vi "CDW_SpecPage.vi"(10 "Spec Page Interface":T2, 11 "MetaDataObj in":refnum<class "MetaDataObj.lvclass">) -> (3 "MetaDataObj out":refnum<class "MetaDataObj.lvclass">)   [LabVIEW 2015, in "NIVS_Consolidated_CDW_MetaDataObj.lvclass"]
uses:
  NIVS_Consolidated_CDW_MetaDataObj.lvclass
  <resource>/dialog/NewProjectWizard/Spec Page Interface.ctl
  <resource>/dialog/NewProjectWizard/MetaDataObj/MetaDataObj.lvclass
  Template Classes/NIVS_Asynchronous/NIVS_Asynchronous.lvclass
  Template Classes/NIVS_Inline HW Interface (Inline-Async)/NIVS_Inline HW Interface (Inline-Async).lvclass
  Template Classes/NIVS_Inline HW Interface/NIVS_Inline HW Interface.lvclass
  Template Classes/NIVS_Inline Model Interface/NIVS_Inline Model Interface.lvclass
  Template Classes/NIVS_Inline Timing and Sync/NIVS_Inline Timing and Sync.lvclass
  Template Classes/NIVS_Asynchronous Timing and Sync/NIVS_Asynchronous Timing and Sync.lvclass
  Template Classes/NIVS_CD Template/NIVS_CD Template.lvclass/NIVS_CD Template.ctl
  NIVS_Consolidated_CDW_MetaDataObj.lvclass/NIVS_Consolidated_CDW_MetaDataObj.ctl
  <resource>/dialog/NewProjectWizard/MetaDataObj/MetaDataObj.lvclass/MetaDataObj.ctl
  Execution Mode.ctl
  Template Classes/NIVS_CD Template/Write Max Instances.vi
  Template Classes/NIVS_CD Template/Write Extra Page Names.vi
  Template Classes/NIVS_CD Template/Write Submenu.vi
  Template Classes/NIVS_CD Template/Write Parent Menu.vi
  <resource>/dialog/NewProjectWizard/MetaDataObj/Accessors/Write Project Name.vi
  <resource>/dialog/NewProjectWizard/MetaDataObj/Accessors/Write Project Root.vi
  Template Classes/NIVS_CD Template/NIVS_CD Template.lvclass
panel:
  in  "Inline-Async":bool=TRUE
  in  "Custom Device Execution Mode":T1(ring)=enum."Inline HW Interface"
  in  "Custom Device Name":string
  in  "Project Root":path
  in  "Maximum Custom Device Instances":u32=1 min=1 max=2474 step=1
  in  "Insert Custom Device in submenu":bool
  in  "Parent Menu Name":string
  in  "Custom Device Extra Page Names":string[](array[string])
  # "Advanced Options"
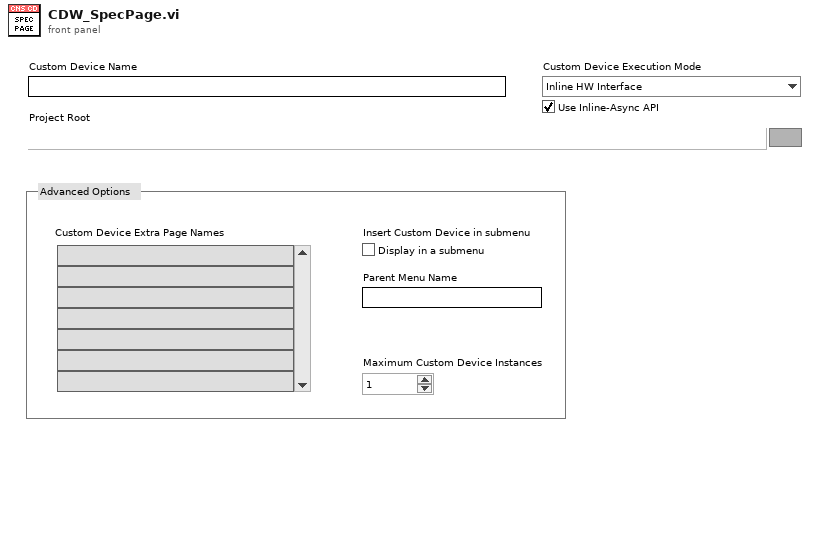
[diagram p1: front panel]
types:
  T1 = enum16{"Asynchronous", "Inline HW Interface", "Inline Model Interface", "Inline Timing and Sync", "Asynchronous Timing and Sync"}
  T2 = typedef "Spec Page Interface.ctl" = cluster{"\"Tab Forward To\" Refnum":refnum<vi>, "\"Tab Backward To\" Refnum":refnum<vi>, "Errors":refnum<user-event>, "Quit":refnum<user-event>}
  T3 = enum8{"Enabled", "Disabled", "Disabled and Grayed Out"}
  T4 = typedef "NIVS_Consolidated_CDW_MetaDataObj.lvclass/Execution Mode.ctl" = enum16{"Asynchronous", "Inline HW Interface", "Inline Model Interface", "Inline Timing and Sync", "Asynchronous Timing and Sync"}
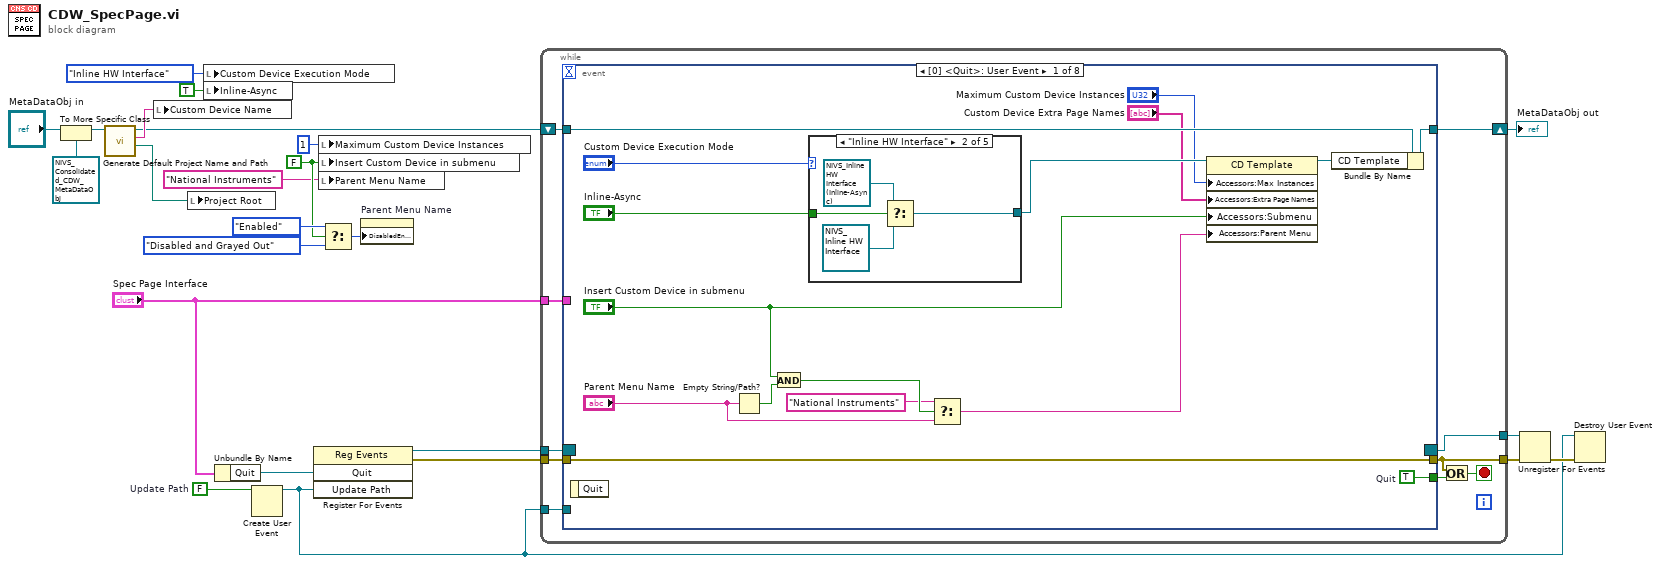
[diagram p0: block diagram]
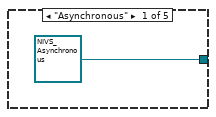
[diagram p2: hidden frame]
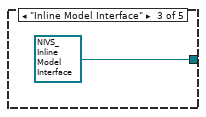
[diagram p3: hidden frame]
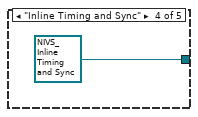
[diagram p4: hidden frame]
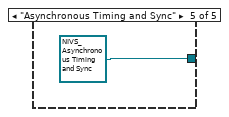
[diagram p5: hidden frame]
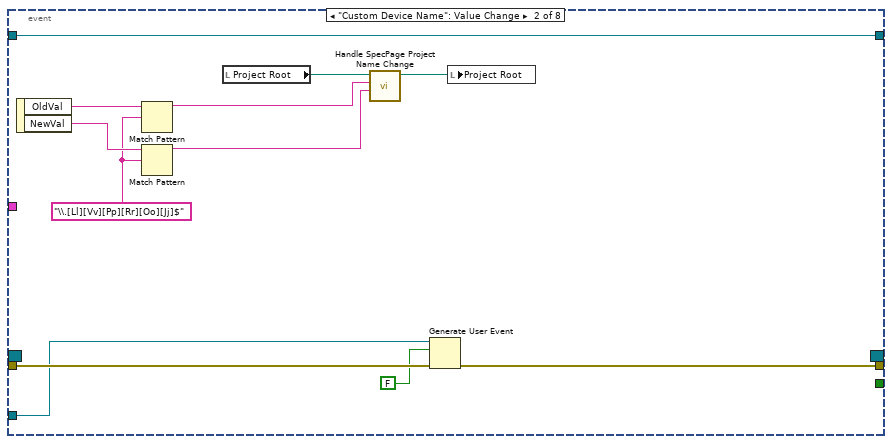
[diagram p6: hidden frame]
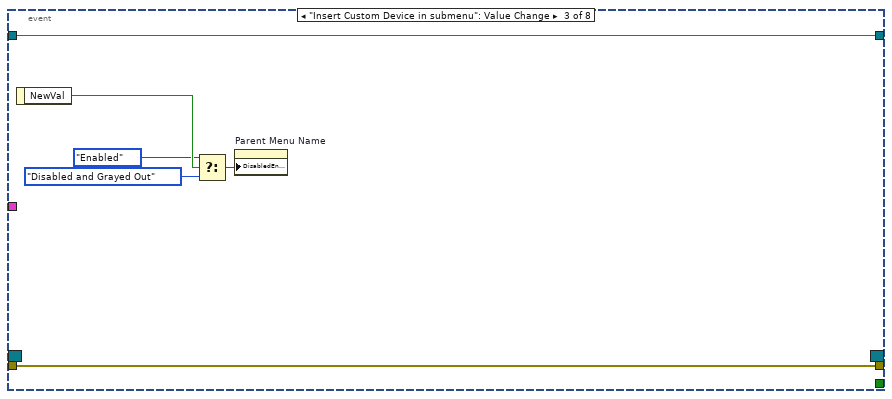
[diagram p7: hidden frame]
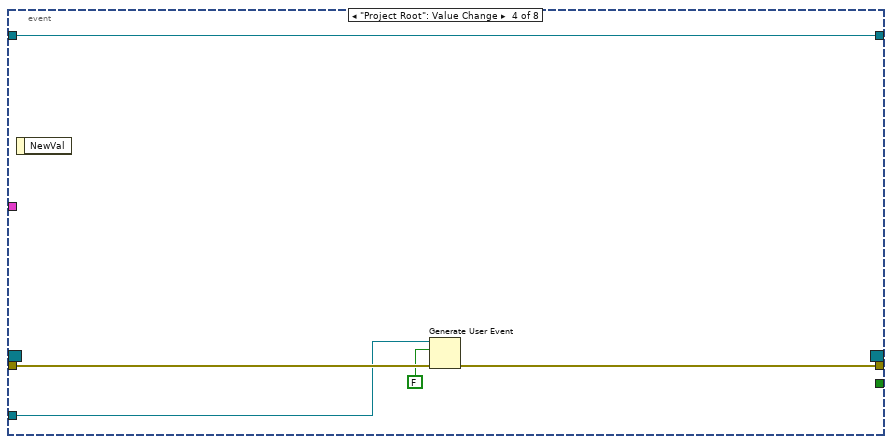
[diagram p8: hidden frame]
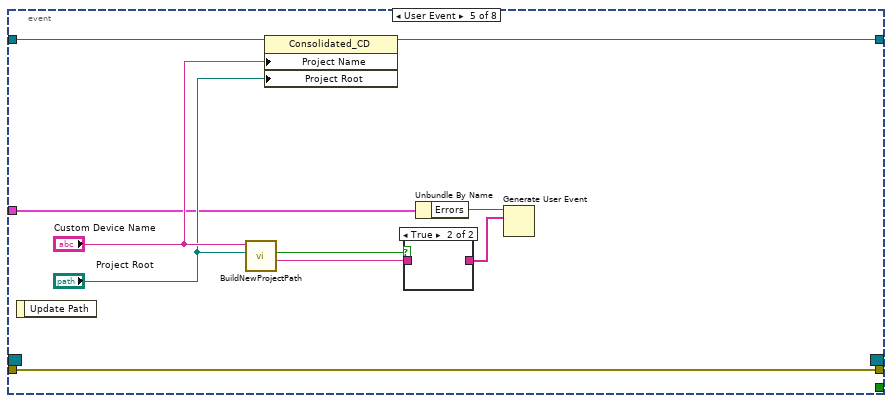
[diagram p9: hidden frame]
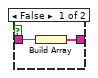
[diagram p10: hidden frame]
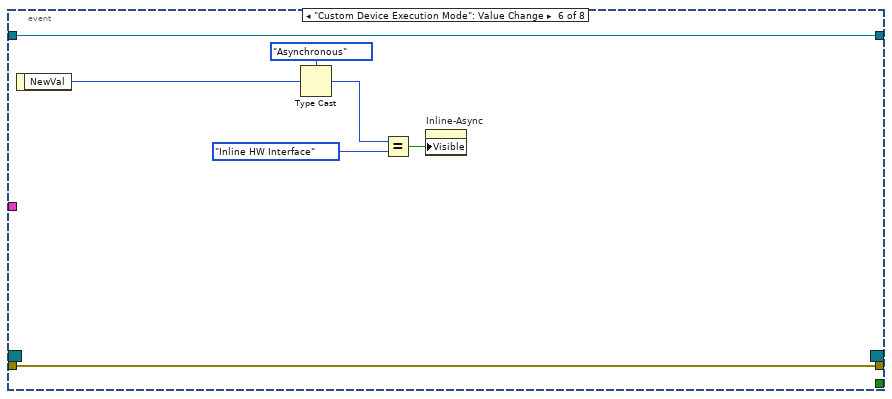
[diagram p11: hidden frame]
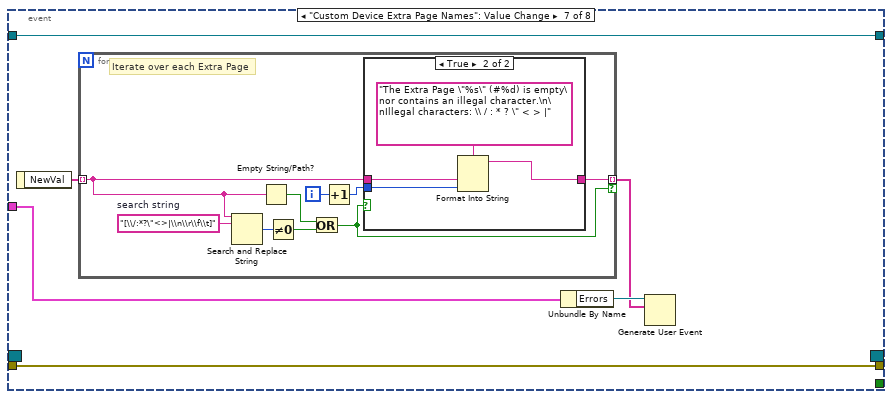
[diagram p12: hidden frame]
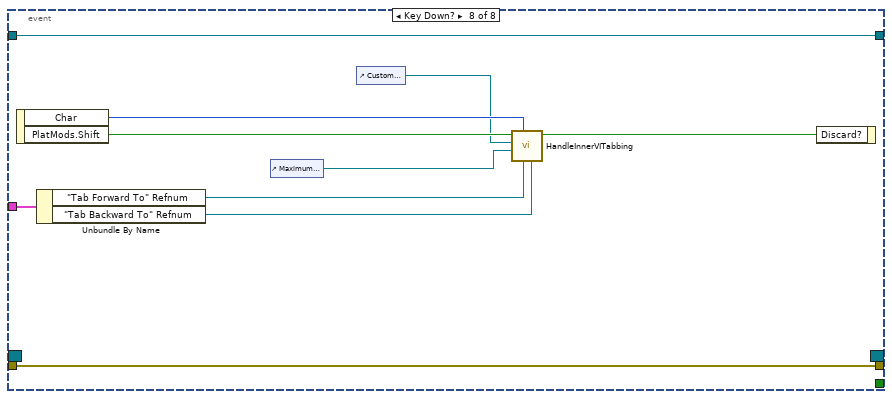
[diagram p14: hidden frame]
diagram:
  w5 = FALSE
  w8 = FALSE  # Update Path
  n1 = To More Specific Class(target class=refnum<class "NIVS_Consolidated_CDW_MetaDataObj.lvclass"> refnum ("Consolidated"), reference="MetaDataObj in") -> (specific class reference=w11:refnum<class "NIVS_Consolidated_CDW_MetaDataObj.lvclass">)  [unwired: 1 in, 1 out]
  n2 = call <resource>:"Generate Default Project Name and Path.vi"("DNL_MetaDataObj in"=w11) -> ("Project Root"=w9:path, "Project Name"=w14:string, "DNL_MetaDataObj out"=w10:refnum<class "NIVS_Consolidated_CDW_MetaDataObj.lvclass">)  [unwired: 8 in]
  n3 = local write "Custom Device Name"(w14) -> ()
  n4 = local write "Project Root"(w9) -> ()
  n5 = local write "Custom Device Execution Mode"(T1."Inline HW Interface" ("Custom Device Execution Mode")) -> ()
  n6 = local write "Inline-Async"(TRUE ("Inline-Async")) -> ()
  n7 = Unbundle By Name("Spec Page Interface") -> ("Quit"=w24:refnum<user-event>)
  n8 = Create User Event(user event datatype=w8) -> (user event=w6:refnum<user-event>)  [unwired: 1 in, 1 out]
  n9 = register-events(w24, w6) -> (reference out=w23:refnum<event-registration>, error out=w19:errorcluster)  [unwired: 2 in]
  n10 = local write "Maximum Custom Device Instances"(u32 1 ("Maximum Custom Device Instances")) -> ()
  n11 = local write "Insert Custom Device in submenu"(w5) -> ()
  n12 = local write "Parent Menu Name"("National Instruments") -> ()
  n13 = Select(t=T3."Enabled" ("Disabled"), s=w5, f=T3."Disabled and Grayed Out") -> (s? t:f=w17:T3)
  n14 = property on="Parent Menu Name" class="Str"("DisabledEnum"=w17) -> ()  [unwired: 2 in, 2 out]
  n15 = while {
    tunnel: "Spec Page Interface" -> [w32]
    shift-right: [w31] -> w20
    shift-left: w10 -> [w30]
    tunnel: w23 -> [w34]
    tunnel: w19 -> [w33]
    tunnel: [w27] -> w21
    tunnel: [w26] -> w13
    tunnel: w6 -> [w25]
    stop <- w29 stop-if-true
    n16 = event shown="[0] <Quit>: User Event" {
      selector: w34 -> [_ _ _ _ _ _ _ _]
      dyn-events: [_ _ _ _ _ _ _ _] -> w26
      timeout: _ -> [_ _ _ _ _ _ _ _]
      tunnel: w32 -> [_ _ _ _ w86 _ w102 w125]
      tunnel: [w50 _ _ _ _ _ _ _] -> w28
      tunnel: [w49 w61 w76 w79 w91 w100 w106 w130] -> w27
      tunnel: w33 -> [w49 w70 w76 w81 w91 w100 w106 w130]
      tunnel: [w47 w69 w75 w80 w89 w99 w104 w129] -> w31
      tunnel: w30 -> [w48 w69 w75 w80 w90 w99 w104 w129]
      tunnel: w25 -> [_ w60 _ w78 _ _ _ _]
      event User Event {
        w50 = TRUE  # Quit
        n17 = event-data() -> ()  [unwired: 1 in, 1 out]
        n18 = Empty String/Path?(string/path="Parent Menu Name") -> (empty?=w45:bool)
        n19 = And(x="Insert Custom Device in submenu", y=w45) -> (x .and. y?=w44:bool)
        n20 = case shown="\"Inline HW Interface\"" "Custom Device Execution Mode" {
          tunnel: "Inline-Async" -> [_ w55 _ _ _]
          tunnel: [refnum<class "NIVS_Asynchronous.lvclass"> refnum ("NIVS_Asynchronous.lvclass") w52 refnum<class "NIVS_Inline Model Interface.lvclass"> refnum ("NIVS_Inline Model Interface.lvclass") refnum<class "NIVS_Inline Timing and Sync.lvclass"> refnum ("NIVS_Inline Timing and Sync.lvclass") refnum<class "NIVS_Asynchronous Timing and Sync.lvclass"> refnum ("NIVS_Asynchronous Timing and Sync.lvclass")] -> w39
          frame "Asynchronous" {
          }
          frame "Inline HW Interface" {
            n21 = Select(t=refnum<class "NIVS_Inline HW Interface (Inline-Async).lvclass"> refnum ("NIVS_Inline HW Interface (Inline-Async).lvclass"), s=w55, f=refnum<class "NIVS_Inline HW Interface.lvclass"> refnum ("NIVS_Inline HW Interface.lvclass")) -> (s? t:f=w52:refnum<class "NIVS_CD Template.lvclass">)
          }
          frame "Inline Model Interface" {
          }
          frame "Inline Timing and Sync" {
          }
          frame "Asynchronous Timing and Sync" {
          }
        }
        n22 = Select(t="National Instruments", s=w44, f="Parent Menu Name") -> (s? t:f=w35:string)
        n23 = property class="CD Template"(reference=w39, "Accessors:Max Instances"="Maximum Custom Device Instances", "Accessors:Extra Page Names"="Custom Device Extra Page Names", "Accessors:Submenu"="Insert Custom Device in submenu", "Accessors:Parent Menu"=w35) -> (reference out=w40:refnum<class "NIVS_CD Template.lvclass">)  [unwired: 1 in, 1 out]
        n24 = Bundle By Name(cluster=w48, "CD Template"=w40) -> (w47:refnum<class "NIVS_Consolidated_CDW_MetaDataObj.lvclass">)
      }
      event "Custom Device Name": Value Change {
        w66 = "\\.[Ll][Vv][Pp][Rr][Oo][Jj]$"
        n25 = event-data() -> ("OldVal"=w68:string, "NewVal"=w67:string)  [unwired: 1 in]
        n26 = Match Pattern(string=w68, regular expression=w66) -> (before substring=w63:string)  [unwired: 1 in, 3 out]
        n27 = Match Pattern(string=w67, regular expression=w66) -> (before substring=w62:string)  [unwired: 1 in, 3 out]
        n28 = local read "Project Root"() -> (w65:path)
        n29 = call <resource>:"Handle SpecPage Project Name Change.vi"("Project Name New Value"=w62, "Project Name Old Value"=w63, "Project Root in"=w65) -> ("Project Root out"=w64:path)  [unwired: 8 in]
        n30 = Generate User Event(user event=w60, event data cluster=FALSE, error in=w70) -> (error out=w61:errorcluster)  [unwired: 1 in, 1 out]
        n31 = local write "Project Root"(w64) -> ()
      }
      event "Insert Custom Device in submenu": Value Change {
        n32 = event-data() -> ("NewVal"=w74:bool)  [unwired: 1 in]
        n33 = Select(t=T3."Enabled" ("Disabled"), s=w74, f=T3."Disabled and Grayed Out") -> (s? t:f=w71:T3)
        n34 = property on="Parent Menu Name" class="Str"("DisabledEnum"=w71) -> ()  [unwired: 2 in, 2 out]
      }
      event "Project Root": Value Change {
        n35 = event-data() -> ()  [unwired: 1 in, 1 out]
        n36 = Generate User Event(user event=w78, event data cluster=FALSE, error in=w81) -> (error out=w79:errorcluster)  [unwired: 1 in, 1 out]
      }
      event User Event {
        n37 = event-data() -> ()  [unwired: 1 in, 1 out]
        n38 = call <resource>:"BuildNewProjectPath.vi"("Project Root"="Project Root", "Project Name"="Custom Device Name") -> ("Error Message"=w85:string, "Valid?"=w82:bool)  [unwired: 7 in, 1 out]
        n39 = property class="Consolidated_CD"(reference=w90, "Project Name"="Custom Device Name", "Project Root"="Project Root") -> (reference out=w89:refnum<class "NIVS_Consolidated_CDW_MetaDataObj.lvclass">)  [unwired: 1 in, 1 out]
        n40 = case shown="True" w82 {
          tunnel: w85 -> [w93 _]
          tunnel: [w92 _] -> w83
          frame False {
            n41 = Build Array(w93) -> (w92:string[])
          }
          frame True {
          }
        }
        n42 = Unbundle By Name(w86) -> ("Errors"=w84:refnum<user-event>)
        n43 = Generate User Event(user event=w84, event data cluster=w83) -> ()  [unwired: 2 in, 2 out]
      }
      event "Custom Device Execution Mode": Value Change {
        n44 = event-data() -> ("NewVal"=w98:T1)  [unwired: 1 in]
        n45 = Type Cast(type=Execution_Mode."Asynchronous" ("CD Wizard - Internal Data.Common Information.CD Execution Mode"), x=w98) -> (*(type *) &x=w96:T4)
        n46 = Equal?(x=w96, y=Execution_Mode."Inline HW Interface") -> (x = y?=w94:bool)
        n47 = property on="Inline-Async" class="Bool (strict)"("Visible"=w94) -> ()  [unwired: 2 in, 2 out]
      }
      event "Custom Device Extra Page Names": Value Change {
        n48 = event-data() -> ("NewVal"=w105:string[])  [unwired: 1 in]
        n49 = for {
          tunnel: w105 -> [w109] mode=indexing
          tunnel: [w108] -> w101 mode=indexing if=w107
          i -> [w111]
          w115 = "[\\/:*?\"<>|\\n\\r\\f\\t]"  # search string
          # "Iterate over each Extra Page"
          n50 = Search and Replace String(input string=w109, search string=w115) -> (number of replacements=w114:i32)  [unwired: 6 in, 3 out]
          n51 = Empty String/Path?(string/path=w109) -> (empty?=w113:bool)
          n52 = Not Equal To 0?(x=w114) -> (x != 0?=w112:bool)
          n53 = Or(x=w113, y=w112) -> (x .or. y?=w107:bool)
          n54 = Increment(x=w111) -> (x+1=w110:i32)
          n55 = case shown="True" w107 {
            tunnel: w110 -> [_ w118]
            tunnel: w109 -> [w116 w119]
            tunnel: [w116 w117] -> w108
            frame False {
              # "Extra Page Name is OK"
            }
            frame True {
              n56 = Format Into String(format string="The Extra Page \"%s\" (#%d) is empty\nor contains an illegal character.\n\nIllegal characters: \\ / : * ? \" < > |", w119, w118) -> (resulting string=w117:string)  [unwired: 2 in, 1 out]
            }
          }
        }
        n57 = Unbundle By Name(w102) -> ("Errors"=w103:refnum<user-event>)
        n58 = Generate User Event(user event=w103, event data cluster=w101) -> ()  [unwired: 2 in, 2 out]
      }
      event Key Down? {
        n59 = event-data() -> ("Char"=w128:i16, "PlatMods.Shift"=w127:bool)  [unwired: 1 in]
        n60 = Unbundle By Name(w125) -> ("\"Tab Forward To\" Refnum"=w124:refnum<vi>, "\"Tab Backward To\" Refnum"=w123:refnum<vi>)
        n61 = control-ref of="Maximum Custom Device Instances"() -> (w121:refnum<vi>)
        n62 = control-ref of="Custom Device Name"() -> (w122:refnum<vi>)
        n63 = call <resource>:"HandleInnerVITabbing.vi"("Tab Backward To"=w123, "Tab Forward To"=w124, "Char"=w128, "Last Control"=w121, "First Control"=w122, "Shift"=w127) -> ("Discard"=w126:bool)  [unwired: 5 in]
        n64 = event-data("Discard?"=w126) -> ()  [unwired: 1 in, 1 out]
      }
    }
    n65 = Or(x=w27, y=w28) -> (x .or. y?=w29:bool)
  }
  "MetaDataObj out" <- w20
  n66 = Unregister For Events(event registration refnum=w13, error in=w21) -> (error out=w7:errorcluster)
  n67 = Destroy User Event(user event=w6, error in=w7) -> ()  [unwired: 1 out]
